vi "util_create_diff_taps.vi"(8 "nfilts":i32, 11 "taps":dbl[](array[numeric])) -> (0 "ntaps":i32, 2 "out diff taps":dbl[][](array[numeric]), 3 "out taps":dbl[][](array[numeric]))   [LabVIEW 2014]
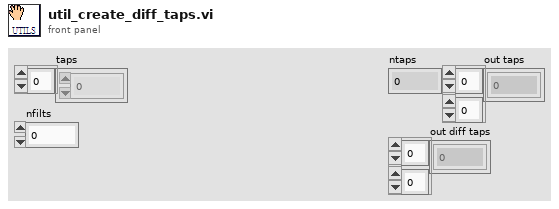
[diagram p1: front panel]
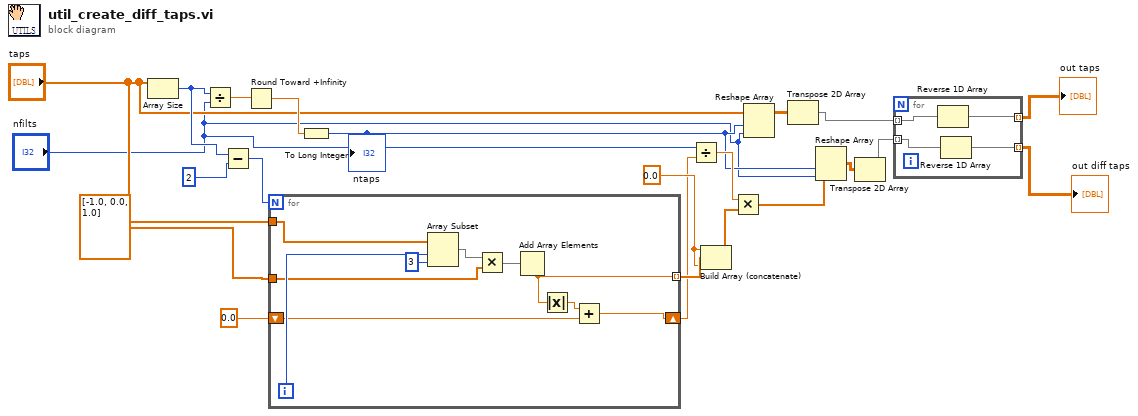
[diagram p0: block diagram]
diagram:
  w13 = 0.0
  n1 = Array Size(array="taps") -> (size(s)=w21:i32)
  n2 = Divide(x=w21, y="nfilts") -> (x/y=w22:dbl)
  n3 = Subtract(x=w21, y=2) -> (x-y=w19:i32)
  n4 = Round Toward +Infinity(x=w22) -> (ceil(x): smallest int >= x=w16:dbl)
  n5 = for {
    N: w19 -> [_]
    tunnel: "taps" -> [w32]
    tunnel: dbl[] [-1.0, 0.0, 1.0] -> [w28]
    tunnel: [w24] -> w14 mode=indexing
    shift-right: [w23] -> w11
    shift-left: 0.0 -> [w25]
    i -> [w31]
    n6 = Array Subset(array=w32, index=w31, length=3) -> (w29:dbl[])
    n7 = Multiply(x=w29, y=w28) -> (x*y=w27:dbl[])
    n8 = Add Array Elements(numeric array=w27) -> (sum=w24:dbl)
    n9 = Absolute Value(x=w24) -> (abs(x)=w26:dbl)
    n10 = Add(x=w26, y=w25) -> (x+y=w23:dbl)
  }
  n11 = To Long Integer(number=w16) -> (32bit integer=w2:i32)
  "ntaps" <- w2
  n12 = Divide(x="nfilts", y=w11) -> (x/y=w10:dbl)
  n13 = Build Array (concatenate)(w13, w14, w13) -> (w12:dbl[])
  n14 = Multiply(x=w10, y=w12) -> (x*y=w9:dbl[])
  n15 = Reshape Array("taps", w2, "nfilts") -> (w6:dbl[][])
  n16 = Transpose 2D Array(2D array=w6) -> (transposed array=w5:dbl[][])
  n17 = Reshape Array(w9, w2, "nfilts") -> (w4:dbl[][])
  n18 = Transpose 2D Array(2D array=w4) -> (transposed array=w3:dbl[][])
  n19 = for {
    tunnel: w5 -> [w36] mode=indexing
    tunnel: w3 -> [w34] mode=indexing
    tunnel: [w35] -> w8 mode=indexing
    tunnel: [w33] -> w7 mode=indexing
    n20 = Reverse 1D Array(array=w36) -> (reversed array=w35:dbl[])
    n21 = Reverse 1D Array(array=w34) -> (reversed array=w33:dbl[])
  }
  "out taps" <- w8
  "out diff taps" <- w7
